vi "Save Test Node.vi"(8 "error in (no error)":errorcluster, 11 "Edit Test Node Model in":refnum<class "Edit Test Node Model.lvclass">) -> (0 "error out":errorcluster, 3 "Edit Test Node Model out":refnum<class "Edit Test Node Model.lvclass">)   [LabVIEW 2013, in "Edit Test Node Model.lvlib" / "Edit Test Node Model.lvclass"]
uses:
  Edit Test Node Model.lvclass
  <vilib>/ActorFramework/Actor/Actor.lvclass/Actor.ctl
  Edit Test Node Model.lvclass/Edit Test Node Model.ctl
  <vilib>/Utility/miscctls.llb/LVPositionTypeDef.ctl
  <vilib>/ActorFrameworkMVC/UI Controller Messages/Move Subpanel Msg/Move Subpanel Msg.lvclass/Move Subpanel Msg.ctl
  <vilib>/ActorFramework/Message Enqueuer/Message Enqueuer.lvclass/Message Enqueuer.ctl
  <vilib>/ActorFrameworkMVC/UI Controller Messages/Insert Subpanel Msg/Insert Subpanel Msg.lvclass/Insert Subpanel Msg.ctl
  <vilib>/ActorFramework/Message Enqueuer/Enqueue.vi
  <vilib>/ActorFramework/Message Priority Queue/Priority Enqueue.vi
  <vilib>/ActorFrameworkMVC/UI Controller Messages/Move Subpanel Msg/Move Subpanel Msg.lvclass
  <vilib>/ActorFrameworkMVC/UI Controller Messages/Insert Subpanel Msg/Insert Subpanel Msg.lvclass
  Test Node Model Messages/Preview Test Node Msg/Preview Test Node Msg.lvclass
  Test Node Model Messages/Update Tiles Info Msg/Update Tiles Info Msg.lvclass
  Test Node Model Messages/Update Previous Button Visibility Msg/Update Previous Button Visibility Msg.lvclass
  Test Node Model Messages/Update Next Button Visibility Msg/Update Next Button Visibility Msg.lvclass
  Common/File IO/File IO.lvlib
  <vilib>/ActorFrameworkMVC/UI Controller Messages/Get Model Actor Enqueuer Msg/Get Model Actor Enqueuer Msg.lvclass
  <vilib>/ActorFramework/Actor/Actor.lvclass
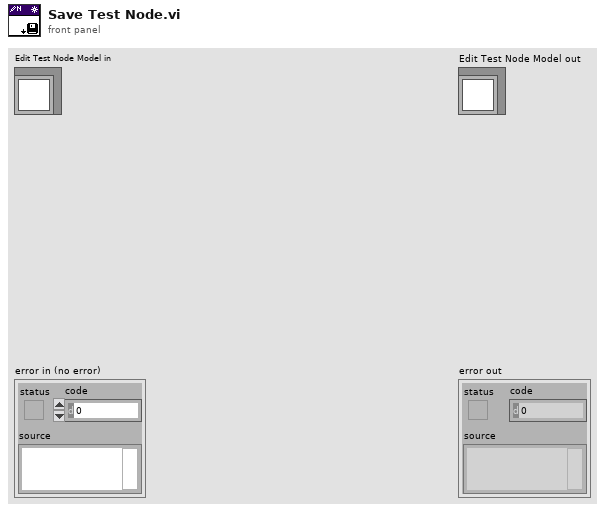
[diagram p1: front panel]
types:
  T1 = typedef "LVPositionTypeDef.ctl" = cluster{"Left":i32, "Top":i32}
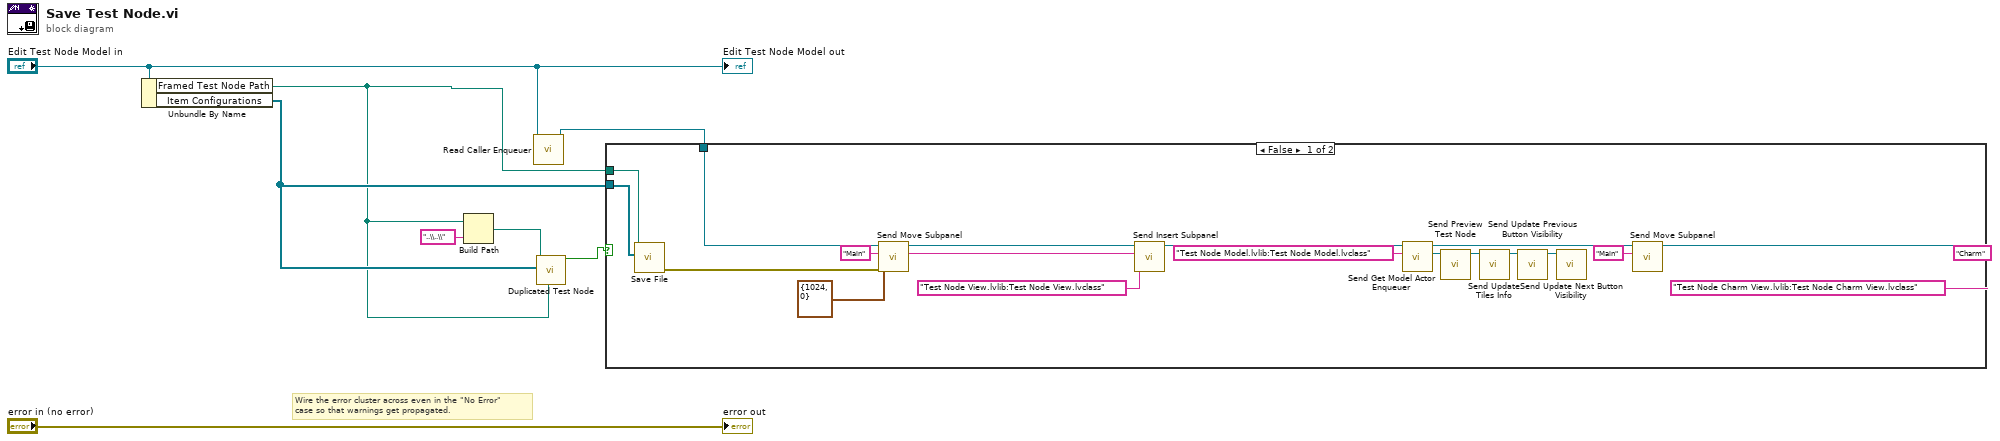
[diagram p0: block diagram]
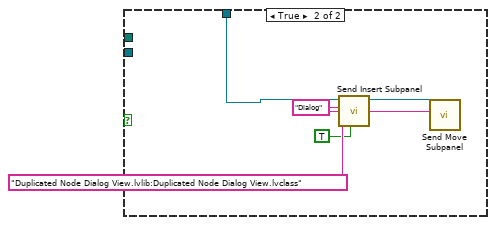
[diagram p2: hidden frame]
diagram:
  # "Wire the error cluster across even in the \"No Error\"\ncase so that warnings get propagated."
  n1 = Unbundle By Name("Edit Test Node Model in") -> ("Framed Test Node Path"=w2:path, "Item Configurations"=w3:refnum<class "Item Configuration.lvclass">[])
  n2 = Build Path(base path=w2, name or relative path="..\\..\\") -> (appended path=w6:path)
  n3 = call <vilib>:"Read Caller Enqueuer.vi"("Actor"="Edit Test Node Model in") -> ("Caller Enqueuer"=w4:refnum<class "Message Enqueuer.lvclass">)  [unwired: 10 in]
  n4 = call "Duplicated Test Node.vi"("Test Node File Path"=w2, "Item Configurations"=w3, "Test Node Directory Path"=w6) -> ("Duplicated?"=w5:bool)  [unwired: 8 in]
  n5 = case shown="False" w5 {
    tunnel: w2 -> [w9 _]
    tunnel: w3 -> [w10 _]
    tunnel: w4 -> [w12 w28]
    frame False {
      w24 = "Main" ("Subpanel Name")
      n6 = call "Save File.vi"("Item Configurations"=w10, "File Path"=w9) -> ("error out"=w11:errorcluster)  [unwired: 9 in]
      n7 = call <vilib>:"Send Move Subpanel.vi"("error in (no error)"=w11, "Position (0,0)"=T1 {"Left"=1024, "Top"=0}, "Subpanel Name"=w24, "Message Enqueuer"=w12) -> ("Message Enqueuer out"=w27:refnum<class "Message Enqueuer.lvclass">)  [unwired: 6 in, 1 out]
      n8 = call <vilib>:"Send Insert Subpanel.vi"("View Name"="Test Node View.lvlib:Test Node View.lvclass" ("Subpanel Name"), "Subpanel Name"=w24, "Message Enqueuer"=w27) -> ("Message Enqueuer out"=w22:refnum<class "Message Enqueuer.lvclass">)  [unwired: 7 in, 1 out]
      n9 = call <vilib>:"Send Get Model Actor Enqueuer.vi"("Model Name"="Test Node Model.lvlib:Test Node Model.lvclass", "Message Enqueuer in"=w22) -> ("Reply"=w13:refnum<class "Message Enqueuer.lvclass">, "Message Enqueuer out"=w21:refnum<class "Message Enqueuer.lvclass">)  [unwired: 6 in, 2 out]
      n10 = call "Send Preview Test Node.vi"("Message Enqueuer"=w13) -> ("Message Enqueuer out"=w19:refnum<class "Message Enqueuer.lvclass">)  [unwired: 9 in, 1 out]
      n11 = call "Send Update Tiles Info.vi"("Message Enqueuer"=w19) -> ("Message Enqueuer out"=w18:refnum<class "Message Enqueuer.lvclass">)  [unwired: 9 in, 1 out]
      n12 = call "Send Update Previous Button Visibility.vi"("Message Enqueuer"=w18) -> ("Message Enqueuer out"=w17:refnum<class "Message Enqueuer.lvclass">)  [unwired: 9 in, 1 out]
      n13 = call "Send Update Next Button Visibility.vi"("Message Enqueuer"=w17) -> ()  [unwired: 9 in, 2 out]
      n14 = call <vilib>:"Send Move Subpanel.vi"("Subpanel Name"="Main", "Message Enqueuer"=w21) -> ("Message Enqueuer out"=w16:refnum<class "Message Enqueuer.lvclass">)  [unwired: 8 in, 1 out]
      n15 = call <vilib>:"Send Insert Subpanel.vi"("View Name"="Test Node Charm View.lvlib:Test Node Charm View.lvclass", "Subpanel Name"="Charm", "Message Enqueuer"=w16) -> ()  [unwired: 7 in, 2 out]
    }
    frame True {
      w30 = "Dialog" ("Subpanel Name")
      n16 = call <vilib>:"Send Insert Subpanel.vi"("Transparent? (F)"=TRUE, "View Name"="Duplicated Node Dialog View.lvlib:Duplicated Node Dialog View.lvclass", "Subpanel Name"=w30, "Message Enqueuer"=w28) -> ("Message Enqueuer out"=w31:refnum<class "Message Enqueuer.lvclass">)  [unwired: 6 in, 1 out]
      n17 = call <vilib>:"Send Move Subpanel.vi"("Subpanel Name"=w30, "Message Enqueuer"=w31) -> ()  [unwired: 8 in, 2 out]
    }
  }
  "error out" <- "error in (no error)"
  "Edit Test Node Model out" <- "Edit Test Node Model in"
